vi "initialize.vi"(8 "error in (no error)":errorcluster) -> (0 "error out":errorcluster)   [LabVIEW 2015, in "lv-waitgroup.lvlib"]
uses:
  lv-waitgroup.lvlib
  private/_controls/fg_command.ctl
  private/_controls/references.ctl
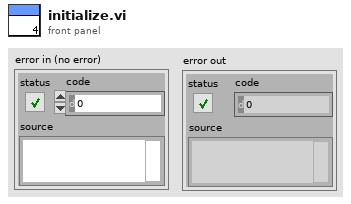
[diagram p1: front panel]
types:
  T1 = typedef "lv-waitgroup.lvlib/references.ctl" = cluster{"waitgroups":refnum<data-value>}
  T2 = typedef "lv-waitgroup.lvlib/fg_command.ctl" = enum16{"<fg_command>", "initialize", "read", "write", "shutdown", "<null>"}
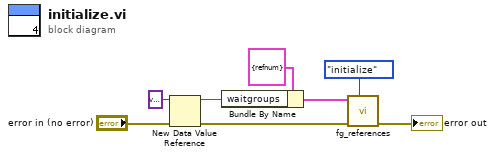
[diagram p0: block diagram]
diagram:
  n1 = New Data Value Reference(data value=variant, error in="error in (no error)") -> (data value reference=w3:refnum<data-value>, error out=w2:errorcluster)
  n2 = Bundle By Name(cluster=T1 {"waitgroups"=refnum} ("references in"), "waitgroups"=w3) -> (w4:T1)
  n3 = call "fg_references.vi"("fg_command"=fg_command."initialize", "error in (no error)"=w2, "references in"=w4) -> ("error out"=→"error out":errorcluster)  [unwired: 7 in, 1 out]
